vi "dfd_Get Structure Groups Relationship.vi"(1 "target group id":T1, 2 "source group id":T1) -> (0 "relationship":i32=-1)   [LabVIEW 2017, in "NI_DigFilterLicensed.lvlib"]
uses:
  <vilib>/addons/Digital Filter Design/NI_DigFilterLicensed.lvlib
  <vilib>/addons/Digital Filter Design/_Objects.llb/DFD Filter Structure Id.ctl
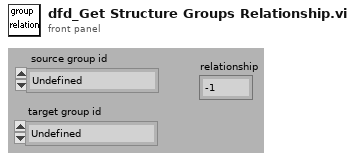
[diagram p1: front panel]
types:
  T1 = typedef "NI_DigFilterLicensed.lvlib/DFD Filter Structure Id.ctl" = enum16{"Undefined", "FIR", "IIR Direct", "IIR SOS", "IIR Allpass", "IIR AR", "IIR ARMA"}
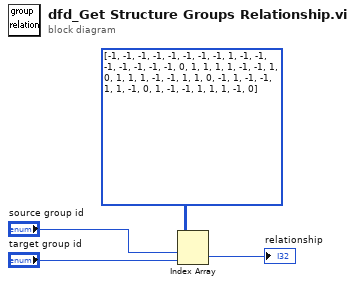
[diagram p0: block diagram]
diagram:
  n1 = Index Array(array=i32[][] [[-1, -1, -1, -1, -1, -1, -1], [-1, 1, -1, -1, -1, -1, -1], [-1, -1, 0, 1, 1, 1, 1], [-1, -1, 1, 0, 1, 1, 1], [-1, -1, 1, 1, 0, -1, 1], [-1, -1, 1, 1, -1, 0, 1], [-1, -1, 1, 1, 1, -1, 0]], index (row)="source group id", index (col)="target group id") -> (element=→"relationship":i32)
